vi "StayOnTarget.vi"() -> ()   [LabVIEW 2020]
panel:
  out "Sum":dbl
  out "QPD 4":dbl
  out "QPD 3":dbl
  out "QPD 2":dbl
  out "QPD 1":dbl
  out "Waveform Chart":dbl(graph)
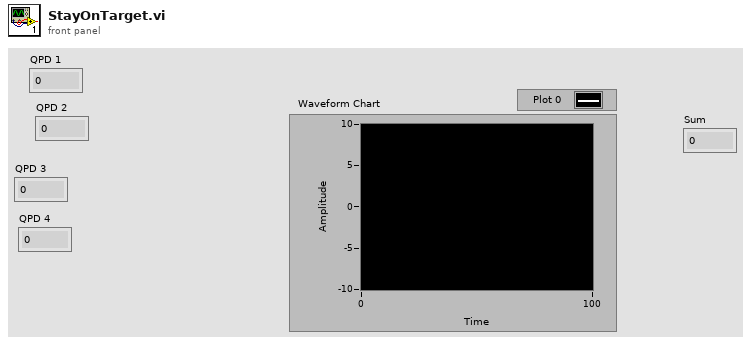
[diagram p1: front panel]
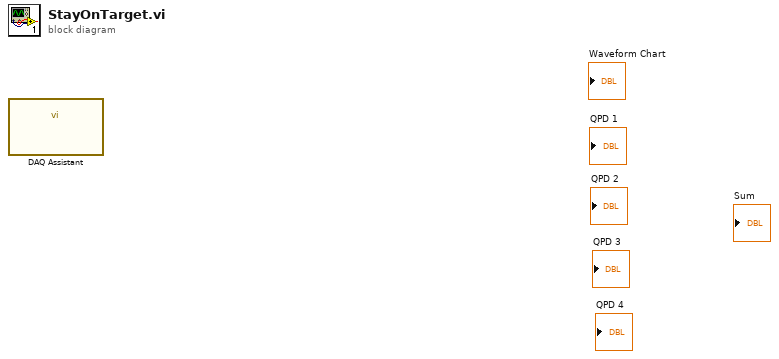
[diagram p0: block diagram]
diagram:
  n1 = call "DAQ Assistant"() -> ()  [unwired: 12 in]
